vi "setAnalogOut.vi"(6 "Value":sgl, 8 "error in (no error)":errorcluster, 9 "PortId":u8, 10 "Device":i32, 11 "SEDSpectrometer in":refnum<class "SEDSpectrometer.lvclass">) -> (0 "error out":errorcluster, 2 "Output Value":i32, 3 "SEDSpectrometer out":refnum<class "SEDSpectrometer.lvclass">)   [LabVIEW 2016, in "SEDSpectrometer.lvclass"]
uses:
  SEDSpectrometer.lvclass
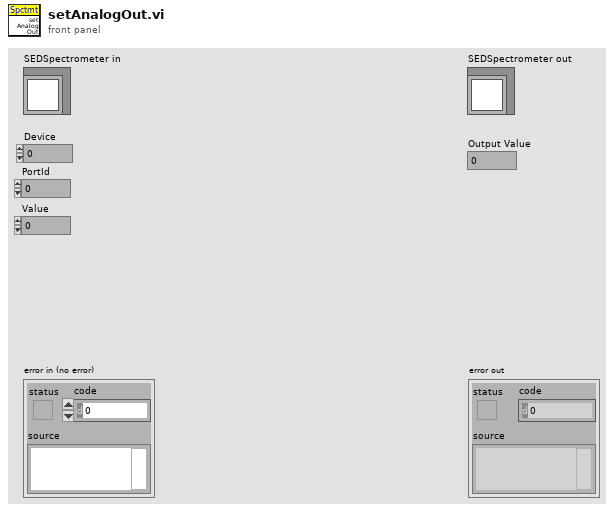
[diagram p1: front panel]
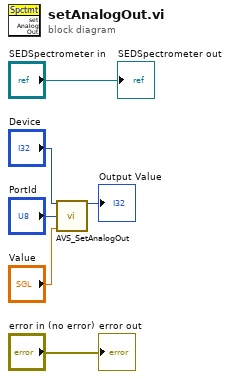
[diagram p0: block diagram]
diagram:
  n1 = call "AVS_SetAnalogOut.vi"("a_hDevice"="Device", "a_PortId"="PortId", "a_Value"="Value") -> ("Output Value"=→"Output Value":i32)  [unwired: 12 in]
  "error out" <- "error in (no error)"
  "SEDSpectrometer out" <- "SEDSpectrometer in"
